vi "PQescapeString.vi"(8 "error in (no error)":errorcluster, 9 "length":u64, 10 "from":string, 11 "to":string) -> (0 "error out":errorcluster, 2 "return type":u64, 3 "to out":string)   [LabVIEW 2019, in "libpqlv64.lvlib"]
uses:
  libpqlv64.lvlib
  libpq.dll
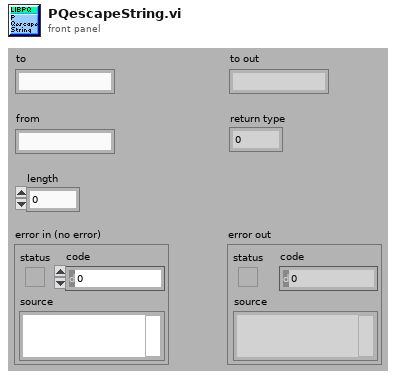
[diagram p1: front panel]
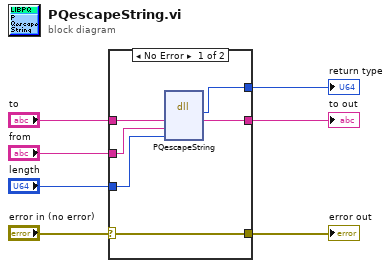
[diagram p0: block diagram]
diagram:
  n1 = case shown="No Error" "error in (no error)" {
    selector: "error in (no error)" -> [w13 w15]
    tunnel: [w13 w15] -> w6
    tunnel: [w12 _] -> w5
    tunnel: "to" -> [w11 w14]
    tunnel: [w10 w14] -> w3
    tunnel: "from" -> [w9 _]
    tunnel: "length" -> [w8 _]
    frame No Error {
      n2 = dll-call lib="libpq.*" fn="PQescapeString"("to"=w11, "from"=w9, "length"=w8) -> ("return type"=w12:u64, "to"=w10:string)  [unwired: 5 in, 2 out]
    }
    frame Error {
    }
  }
  "return type" <- w5
  "to out" <- w3
  "error out" <- w6
